vi "Destroy-Window.vi"(8 "error in (no error)":errorcluster, 11 "GLF Window in":refnum<class "Window.lvclass">) -> (0 "error out":errorcluster)   [LabVIEW 2020, in "GLF.lvlib" / "Window.lvclass"]
uses:
  Window.lvclass
  Window.lvclass/Window.ctl
  IAmGLF/IAmGLF.lvclass
  Engine/Engine.lvclass
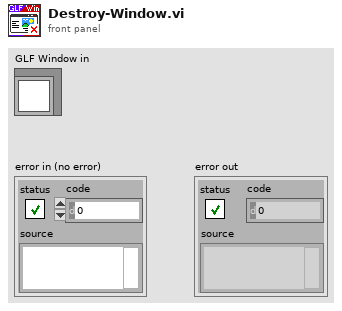
[diagram p1: front panel]
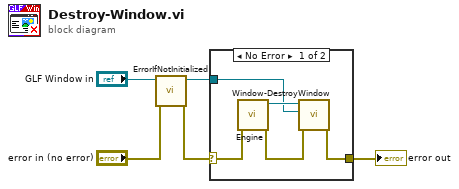
[diagram p0: block diagram]
diagram:
  n1 = call "ErrorIfNotInitialized.vi"("error in (no error)"="error in (no error)", "IAmGLF in"="GLF Window in") -> ("error out"=w3:errorcluster, "IAmGLF out"=w2:refnum<class "Window.lvclass">)  [unwired: 8 in]
  n2 = case shown="No Error" w3 {
    selector: w3 -> [w10 w11]
    tunnel: w2 -> [w8 _]
    tunnel: [w6 w11] -> w1
    frame No Error {
      n3 = call "Engine.vi"("error in (no error)"=w10) -> ("error out"=w7:errorcluster, "Engine"=w9:refnum<class "Engine.lvclass">)  [unwired: 9 in]
      n4 = call "Window-DestroyWindow.vi"("error in (no error)"=w7, "Window Instance"=w8, "Engine in"=w9) -> ("error out"=w6:errorcluster)  [unwired: 7 in, 1 out]
    }
    frame Error {
    }
  }
  "error out" <- w1
